vi "點檢_VI_畫十字線.vi"(8 "error in (no error)":errorcluster, 11 "Refnum in":T1) -> (0 "error out":errorcluster, 2 "中心點":cluster{sgl, sgl}, 3 "Refnum out":T1)   [LabVIEW 2015]
uses:
  <vilib>/vision/Image Controls.llb/IMAQ Image.ctl
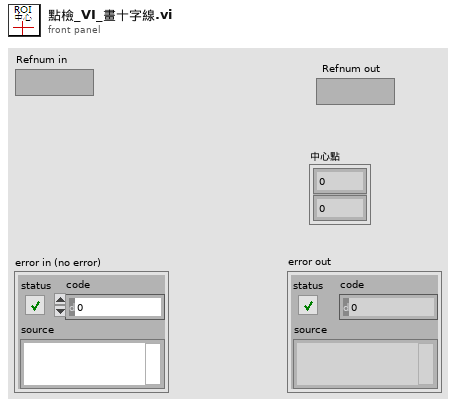
[diagram p1: front panel]
types:
  T1 = typedef "IMAQ Image.ctl" = refnum<image>
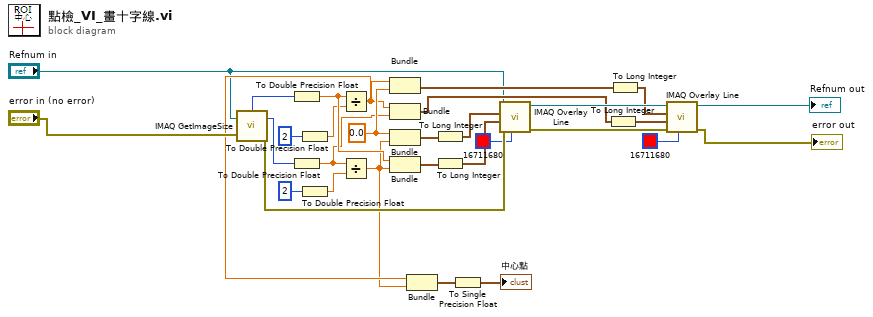
[diagram p0: block diagram]
diagram:
  w22 = 0.0
  n1 = call "IMAQ GetImageSize"("Image"="Refnum in", "error in (no error)"="error in (no error)") -> ("Y Resolution"=w26:i32, "X Resolution"=w5:i32, "error out"=w28:errorcluster)  [unwired: 2 in]
  n2 = To Double Precision Float(number=w5) -> (double precision float=w23:dbl)
  n3 = To Double Precision Float(number=w26) -> (double precision float=w21:dbl)
  n4 = To Double Precision Float(number=2 ("y")) -> (double precision float=w12:dbl)
  n5 = To Double Precision Float(number=2 ("y")) -> (double precision float=w11:dbl)
  n6 = Divide(x=w23, y=w12) -> (x/y=w9:dbl)
  n7 = Divide(x=w21, y=w11) -> (x/y=w8:dbl)
  n8 = Bundle(w9, w22) -> (w20:cluster{dbl, dbl})  [unwired: 1 in]
  n9 = Bundle(w9, w21) -> (w18:cluster{dbl, dbl})  [unwired: 1 in]
  n10 = Bundle(w22, w8) -> (w16:cluster{dbl, dbl})  [unwired: 1 in]
  n11 = Bundle(w23, w8) -> (w14:cluster{dbl, dbl})  [unwired: 1 in]
  n12 = Bundle(w9, w8) -> (w7:cluster{dbl, dbl})  [unwired: 1 in]
  n13 = To Long Integer(number=w16) -> (32bit integer=w15:cluster{i32, i32})
  n14 = To Long Integer(number=w14) -> (32bit integer=w13:cluster{i32, i32})
  n15 = To Single Precision Float(number=w7) -> (single precision float=→"中心點":cluster{sgl, sgl})
  n16 = call "IMAQ Overlay Line"("Color"=u32 16711680, "error in (no error)"=w28, "End Point"=w13, "Start Point"=w15, "Image"="Refnum in") -> ("error out"=w29:errorcluster, "Image Out"=w27:T1)  [unwired: 5 in]
  n17 = To Long Integer(number=w18) -> (32bit integer=w17:cluster{i32, i32})
  n18 = To Long Integer(number=w20) -> (32bit integer=w19:cluster{i32, i32})
  n19 = call "IMAQ Overlay Line"("Color"=u32 16711680, "error in (no error)"=w29, "End Point"=w17, "Start Point"=w19, "Image"=w27) -> ("error out"=→"error out":errorcluster, "Image Out"=→"Refnum out":T1)  [unwired: 5 in]
